vi "Variables Globales.vi"() -> ()   [LabVIEW 2020]
panel:
  in  "Botón de Modo Manual":bool
  out "Luz de ajuste":bool
  out "Llenado completado":bool
  out "Caudal estimado":dbl
  out "dt":dbl
  out "Ciclo de llenado":bool
  out "Peso objetivo actual":dbl
  out "Nivel medido del tanque":dbl
  out "Peso medido del pote de yogurt":dbl
  out "Nivel real del tanque":dbl
  out "Pote de yogurt en la máquina":bool
  out "Modo Manual":bool
  out "Error detectado":bool
  out "Nivel del tanque":dbl
  in  "Botón de Enter":bool
  in  "Boton de emergencia":bool
  in  "Boton de ajuste":bool
  out "% De Apertura de la válvula":dbl
  out "Pantalla LCD":string
  out "Nivel de tanque bajo":bool
  out "Ajuste":bool
  out "Emergencia":bool
  out "Peso real del pote de Yogurt":dbl
  out "Peso objetivo seteado por perilla":dbl
  # "Actuadores"
  # "Indicadores"
  # "Pulsadores"
  # "Variables reales"
  # "Variables medidas"
  # "Settings"
  # "Valores de la simulación"
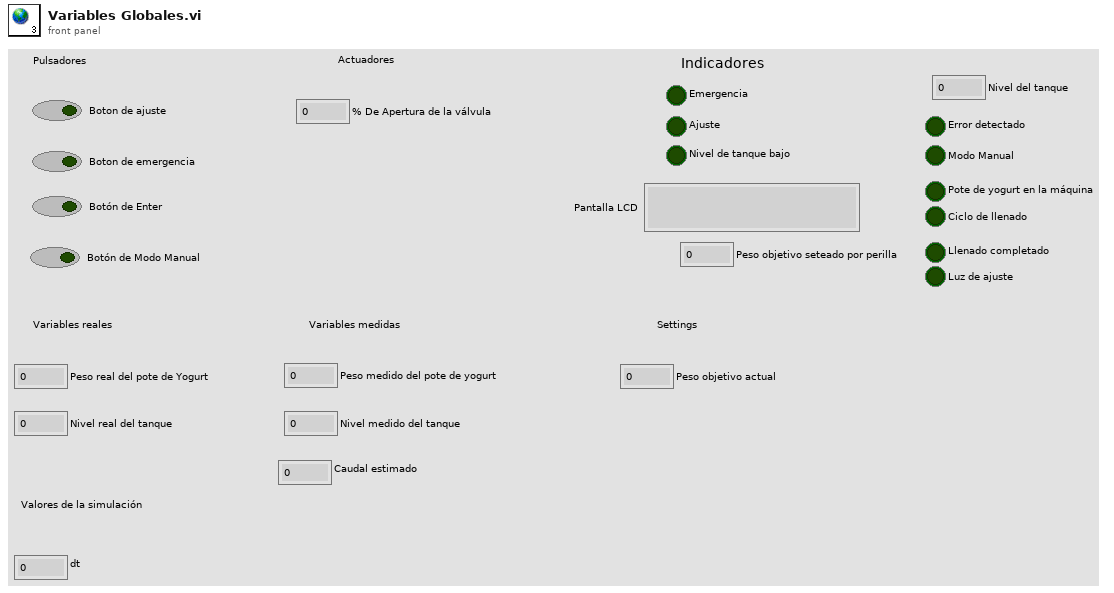
[diagram p1: front panel]
diagram:
